vi "Dynamic Load NI Scope.vi"(8 "Error In":errorcluster, 9 "Debug":bool) -> (0 "Error Out":errorcluster, 2 "Device names":string[](array[string]), 3 "Digitizers out":refnum<class "Pulse Driver.lvclass">[](array[class]))   [LabVIEW 2021]
uses:
  Instruments/Pulse Driver/Pulse Driver.lvclass
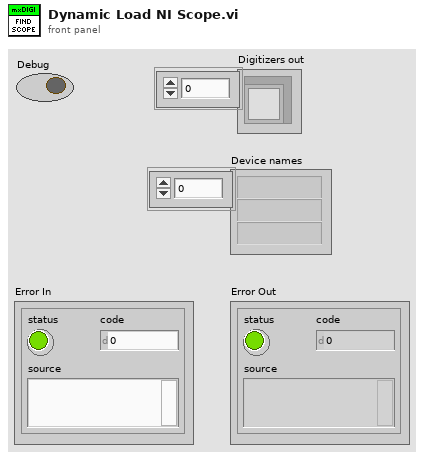
[diagram p1: front panel]
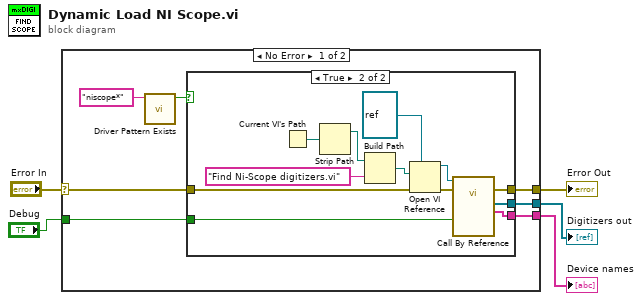
[diagram p0: block diagram]
diagram:
  n1 = case shown="No Error" "Error In" {
    selector: "Error In" -> [w9 w26]
    tunnel: [w12 w26] -> w3
    tunnel: [w11 _] -> w5
    tunnel: [w10 _] -> w4
    tunnel: "Debug" -> [w6 _]
    frame No Error {
      n2 = call "Driver Pattern Exists.vi"("File pattern"="niscope*") -> ("file or folder exists?"=w8:bool)  [unwired: 10 in]
      n3 = case shown="True" w8 {
        tunnel: w9 -> [w13 w20]
        tunnel: [w13 w17] -> w12
        tunnel: [_ w18] -> w11
        tunnel: [_ w15] -> w10
        tunnel: w6 -> [_ w14]
        frame False {
        }
        frame True {
          n4 = Current VI's Path() -> (path=w24:path)
          n5 = Strip Path(path=w24) -> (stripped path=w16:path)  [unwired: 1 out]
          n6 = Build Path(base path=w16, name or relative path="Find Ni-Scope digitizers.vi") -> (appended path=w19:path)
          n7 = Open VI Reference(type specifier VI Refnum (for type only)=refnum<vi> refnum, vi path=w19, error in (no error)=w20) -> (vi reference=w22:refnum<vi>, error out=w21:errorcluster)  [unwired: 3 in]
          n8 = call-by-ref "?"(reference=w22, error in=w21, "Debug"=w14) -> (error out=w17:errorcluster, "Device names out"=w18:string[], "Digitizers out"=w15:refnum<class "Pulse Driver.lvclass">[])  [unwired: 8 in, 2 out]
        }
      }
    }
    frame Error {
    }
  }
  "Error Out" <- w3
  "Digitizers out" <- w4
  "Device names" <- w5
